vi "Create Response.vi"(8 "error in (no error)":errorcluster, 11 "Message Channel in":T1 format="%.0x") -> (0 "error out":errorcluster, 3 "Message Channel out":T1 format="%.0x")   [LabVIEW 2018, in "Instrument Addon Scripting API.lvlib"]
uses:
  Instrument Addon Scripting API.lvlib
  <vilib>/NI Veristand/Custom Device API/Custom Device Item Ref.ctl
  Addon/Addon Shared/SubVIs/Constants.vi
  Addon/Addon Shared/Instrument Addon Shared.lvlib
  <vilib>/NI Veristand/Custom Device API/Custom Device API.lvlib
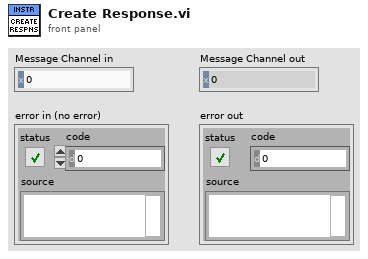
[diagram p1: front panel]
types:
  T1 = typedef "Custom Device API.lvlib/Custom Device Item Ref.ctl" = u64
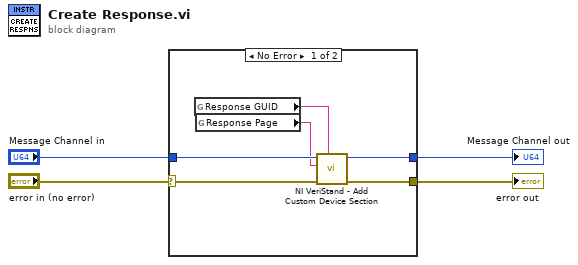
[diagram p0: block diagram]
diagram:
  n1 = case shown="No Error" "error in (no error)" {
    selector: "error in (no error)" -> [w5 w11]
    tunnel: [w10 w12] -> w4
    tunnel: [w9 w11] -> w3
    tunnel: "Message Channel in" -> [w8 w12]
    frame No Error {
      n2 = global read "Constants.vi" "Response GUID"() -> (w7:string)
      n3 = global read "Constants.vi" "Response Page"() -> (w6:string)
      n4 = call <vilib>:"NI VeriStand - Add Custom Device Section.vi"("GUID (Default Section)"=w7, "error in (no error)"=w5, "Section Name"=w6, "Parent Ref in"=w8) -> ("error out"=w9:errorcluster, "Parent Ref out"=w10:T1)  [unwired: 4 in, 2 out]
    }
    frame Error {
    }
  }
  "Message Channel out" <- w4
  "error out" <- w3
